vi "Is Available.vi"(8 "error in (no error)":errorcluster, 11 "Test Framework in":refnum<class "Test Framework.lvclass">) -> (0 "error out":errorcluster, 2 "Is Available":bool, 3 "Test Framework out":refnum<class "Test Framework.lvclass">)   [LabVIEW 2017, in "Framework.lvlib" / "Test Framework.lvclass"]
doc: "Indicates whether the test framework is currently available. This method must not directly link to the test framework."
uses:
  Test Framework.lvclass
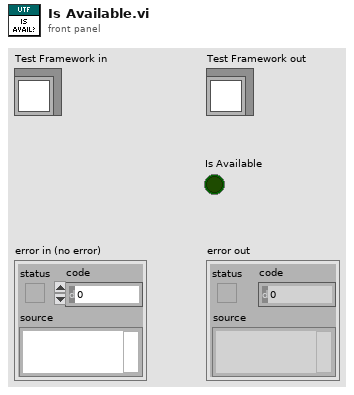
[diagram p1: front panel]
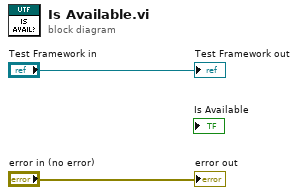
[diagram p0: block diagram]
diagram:
  "error out" <- "error in (no error)"
  "Test Framework out" <- "Test Framework in"
